vi "RT Loop Timer.vi"(8 "start time":u32, 10 "loop counter":i32) -> (0 "RT loop rate (kHz)":dbl=21894.0 format="%#.3g", 2 "RT Loop Rate (ms)":u32=2)   [LabVIEW 2018]
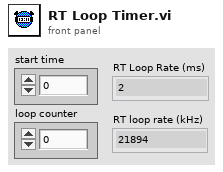
[diagram p1: front panel]
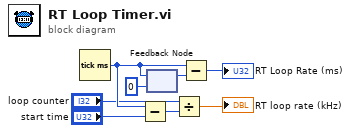
[diagram p0: block diagram]
diagram:
  n1 = Tick Count (ms)() -> (millisecond timer value=w4:u32)
  n2 = Subtract(x=w4, y="start time") -> (x-y=w3:u32)
  n3 = feedback #1(u32 0 ("millisecond timer value")) -> (w7:u32)
  n4 = feedback-in #1(w4) -> ()
  n5 = Divide(x="loop counter", y=w3) -> (x/y=→"RT loop rate (kHz)":dbl)
  n6 = Subtract(x=w4, y=w7) -> (x-y=→"RT Loop Rate (ms)":u32)
